vi "Elaborazione Potenze.vi"(4 "Np_Analysis":i32, 5 "Cluster":T1) -> (0 "transposed array":dbl[][](array[numeric]), 1 "fs - Detected frequency \nof the signal":dbl format="%.2p")   [LabVIEW 2018]
uses:
  coppie.ctl
  array misure.ctl
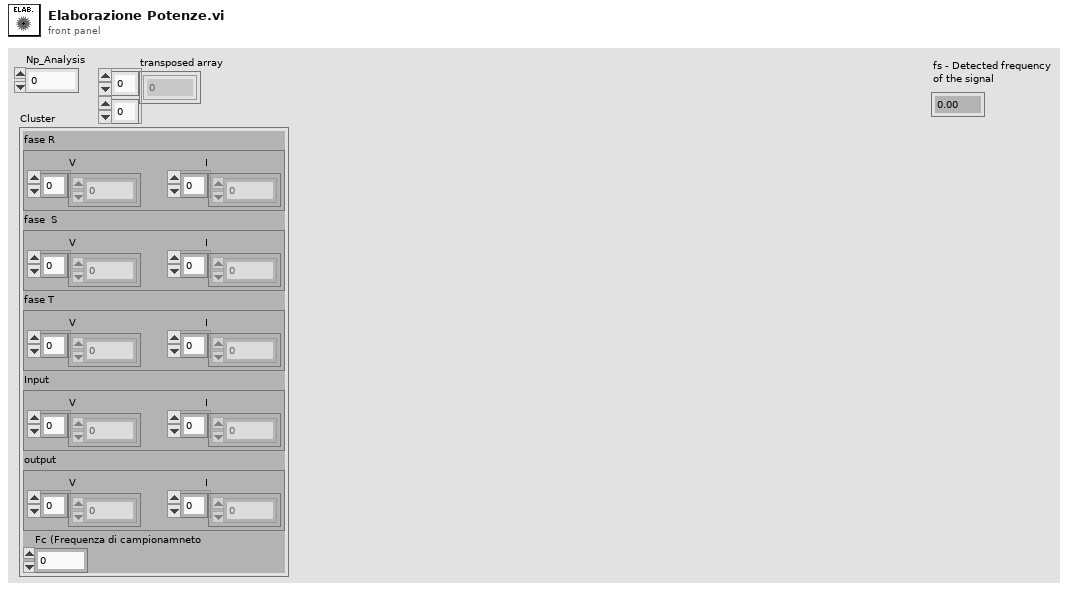
[diagram p1: front panel]
types:
  T1 = typedef "array misure.ctl" = cluster{"fase R ":T2, "fase  S":T2, "fase T":T2, "Input":T2, "output":T2, "Fc (Frequenza di campionamneto":dbl}
  T2 = typedef "coppie.ctl" = cluster{"V":dbl[], "I":dbl[]}
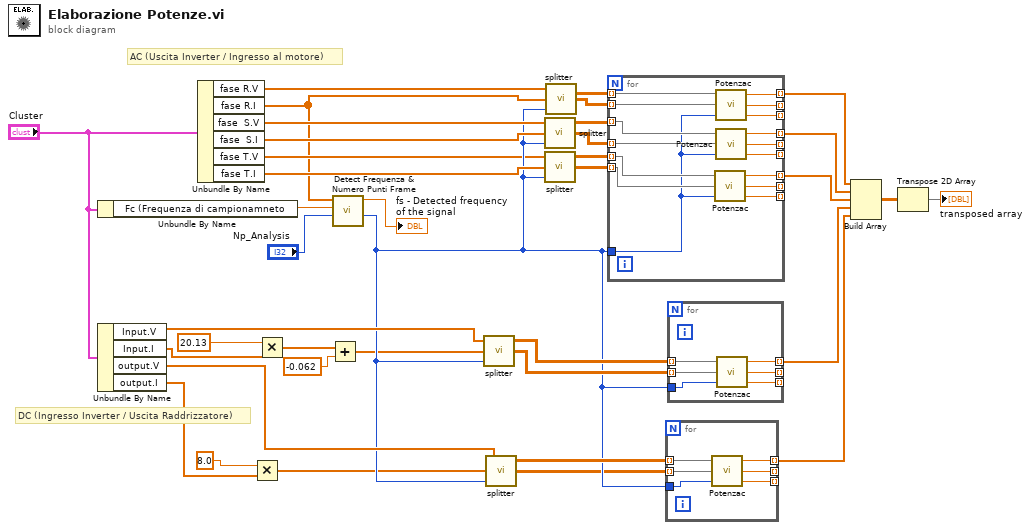
[diagram p0: block diagram]
diagram:
  # "DC (Ingresso Inverter / Uscita Raddrizzatore)"
  # "AC (Uscita Inverter / Ingresso al motore)"
  n1 = Unbundle By Name("Cluster") -> ("Fc (Frequenza di campionamneto"=w36:dbl)
  n2 = Unbundle By Name("Cluster") -> ("Input.V"=w24:dbl[], "Input.I"=w23:dbl[], "output.V"=w20:dbl[], "output.I"=w2:dbl[])
  n3 = Unbundle By Name("Cluster") -> ("fase R.V"=w34:dbl[], "fase R.I"=w16:dbl[], "fase  S.V"=w31:dbl[], "fase  S.I"=w30:dbl[], "fase T.V"=w17:dbl[], "fase T.I"=w27:dbl[])
  n4 = Multiply(x=8.0, y=w2) -> (x*y=w1:dbl[])
  n5 = Multiply(x=20.13, y=w23) -> (x*y=w8:dbl[])
  n6 = Add(x=w8, y=-0.062) -> (x+y=w6:dbl[])
  n7 = call "Detect Frequenza & Numero Punti Frame.vi"("Np_Analysis"="Np_Analysis", "fc - Sampling frequency \nof the card"=w36, "Signal"=w16) -> ("Npp_Frame"=w18:i32, "fs - Detected frequency \nof the signal"=→"fs - Detected frequency \nof the signal":dbl)  [unwired: 7 in]
  n8 = call "splitter.vi"("Npp_Frame"=w18, "Current"=w6, "Voltage"=w24) -> ("Current Array"=w21:dbl[][], "Voltage Array"=w22:dbl[][])  [unwired: 1 in]
  n9 = call "splitter.vi"("Npp_Frame"=w18, "Current"=w1, "Voltage"=w20) -> ("Current Array"=w4:dbl[][], "Voltage Array"=w19:dbl[][])  [unwired: 1 in]
  n10 = call "splitter.vi"("Npp_Frame"=w18, "Current"=w30, "Voltage"=w31) -> ("Current Array"=w28:dbl[][], "Voltage Array"=w29:dbl[][])  [unwired: 1 in]
  n11 = call "splitter.vi"("Npp_Frame"=w18, "Current"=w27, "Voltage"=w17) -> ("Current Array"=w25:dbl[][], "Voltage Array"=w26:dbl[][])  [unwired: 1 in]
  n12 = call "splitter.vi"("Npp_Frame"=w18, "Current"=w16, "Voltage"=w34) -> ("Current Array"=w32:dbl[][], "Voltage Array"=w33:dbl[][])  [unwired: 1 in]
  n13 = for {
    tunnel: w33 -> [w54] mode=indexing
    tunnel: w32 -> [w53] mode=indexing
    tunnel: w18 -> [w46]
    tunnel: [w52] -> w15 mode=indexing
    tunnel: [w51] -> _ mode=indexing
    tunnel: w29 -> [w50] mode=indexing
    tunnel: w28 -> [w49] mode=indexing
    tunnel: w26 -> [w48] mode=indexing
    tunnel: w25 -> [w47] mode=indexing
    tunnel: [w45] -> w14 mode=indexing
    tunnel: [w44] -> _ mode=indexing
    tunnel: [w43] -> _ mode=indexing
    tunnel: [w42] -> _ mode=indexing
    tunnel: [w41] -> w13 mode=indexing
    tunnel: [w40] -> _ mode=indexing
    tunnel: [w39] -> _ mode=indexing
    n14 = call "Potenzac.vi"("Npp_Frame"=w46, "I"=w47, "V"=w48) -> ("Apparent Power"=w39:dbl, "Reactive Power"=w40:dbl, "Active Power"=w41:dbl)
    n15 = call "Potenzac.vi"("Npp_Frame"=w46, "I"=w53, "V"=w54) -> ("Apparent Power"=w43:dbl, "Reactive Power"=w51:dbl, "Active Power"=w52:dbl)
    n16 = call "Potenzac.vi"("Npp_Frame"=w46, "I"=w49, "V"=w50) -> ("Apparent Power"=w42:dbl, "Reactive Power"=w44:dbl, "Active Power"=w45:dbl)
  }
  n17 = for {
    tunnel: w19 -> [w60] mode=indexing
    tunnel: w4 -> [w59] mode=indexing
    tunnel: w18 -> [w58]
    tunnel: [w57] -> w11 mode=indexing
    tunnel: [w56] -> _ mode=indexing
    tunnel: [w55] -> _ mode=indexing
    n18 = call "Potenzac.vi"("Npp_Frame"=w58, "I"=w59, "V"=w60) -> ("Apparent Power"=w55:dbl, "Reactive Power"=w56:dbl, "Active Power"=w57:dbl)
  }
  n19 = for {
    tunnel: w22 -> [w66] mode=indexing
    tunnel: w21 -> [w65] mode=indexing
    tunnel: w18 -> [w64]
    tunnel: [w63] -> w12 mode=indexing
    tunnel: [w62] -> _ mode=indexing
    tunnel: [w61] -> _ mode=indexing
    n20 = call "Potenzac.vi"("Npp_Frame"=w64, "I"=w65, "V"=w66) -> ("Apparent Power"=w61:dbl, "Reactive Power"=w62:dbl, "Active Power"=w63:dbl)
  }
  n21 = Build Array(w15, w14, w13, w12, w11) -> (w10:dbl[][])
  n22 = Transpose 2D Array(2D array=w10) -> (transposed array=→"transposed array":dbl[][])
